vi "SetDAC_04.vi"(0 "RS232/ Optical Fiber":refnum<visa-resource-name>="COM2", 1 "DATA (V)":dbl min=-5000.0 max=5000.0 step=0.001 format="%.2f", 2 "DAC nr":u8=1, 3 "All to zero":bool, 4 "DAC write (mV)":dbl[](array[numeric]) min=-2000.0 max=2000.0) -> (5 "DAC read (mV)":dbl[](array[numeric]))   [LabVIEW 2011]
uses:
  DACreadglobal.vi
panel:
  # "Dilution room :  COM2"
  # "Set dac value manually\nDac values are swept safely"
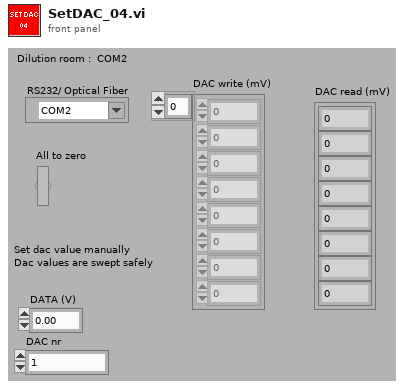
[diagram p1: front panel]
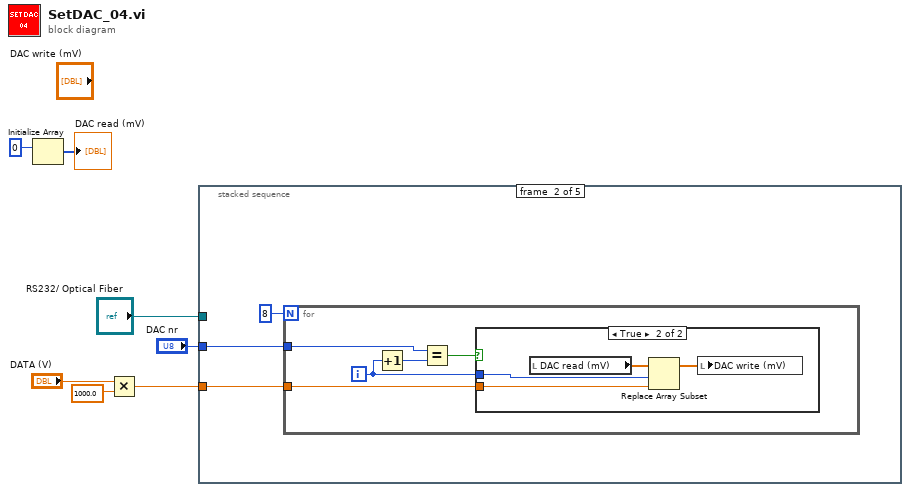
[diagram p0: block diagram]
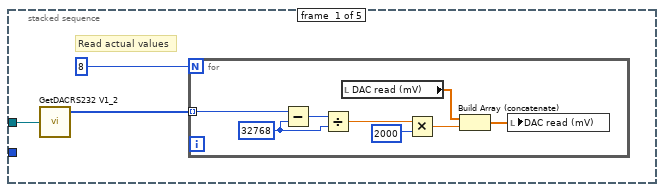
[diagram p2: hidden frame]
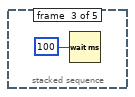
[diagram p4: hidden frame]
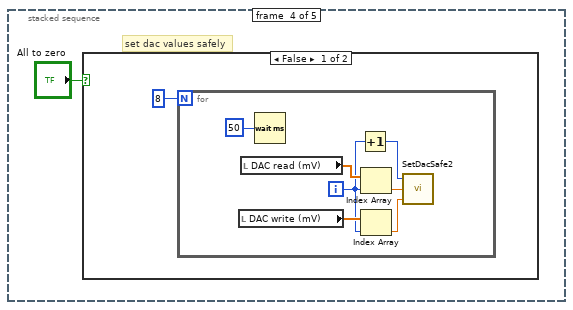
[diagram p5: hidden frame]
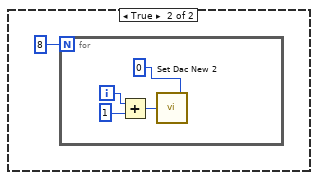
[diagram p6: hidden frame]
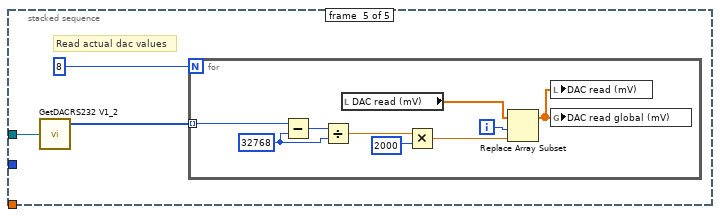
[diagram p7: hidden frame]
diagram:
  n1 = Initialize Array(0) -> (→"DAC read (mV)":i32[])  [unwired: 1 in]
  n2 = Multiply(x="DATA (V)", y=1000.0) -> (x*y=w1:dbl)
  n3 = stacked-sequence {
    tunnel: "RS232/ Optical Fiber" -> [w10 _ _ _ w48]
    tunnel: "DAC nr" -> [_ w20 _ _ _]
    tunnel: w1 -> [_ w19 _ _ _]
    frame #0 {
      # "Read actual values"
      n4 = call "GetDACRS232 V1_2.vi"("VISA resource name IN"=w10) -> ("DAC data out\n(hexadecimaal)"=w8:u16[])  [unwired: 2 in, 2 out]
      n5 = for {
        N: 8 -> [_]
        tunnel: w8 -> [w14] mode=indexing
        w17 = 32768
        n6 = Subtract(x=w14, y=w17) -> (x-y=w18:i32)
        n7 = Divide(x=w18, y=w17) -> (x/y=w16:dbl)
        n8 = local read "DAC read (mV)"() -> (w13:dbl[])
        n9 = Multiply(x=w16, y=2000) -> (x*y=w11:dbl)
        n10 = Build Array (concatenate)(w13, w11) -> (w12:dbl[])
        n11 = local write "DAC read (mV)"(w12) -> ()
      }
    }
    frame #1 {
      n12 = for {
        N: 8 -> [_]
        tunnel: w20 -> [w25]
        tunnel: w19 -> [w22]
        i -> [w23]
        n13 = Increment(x=w23) -> (x+1=w26:i32)
        n14 = Equal?(x=w25, y=w26) -> (x = y?=w24:bool)
        n15 = case shown="True" w24 {
          tunnel: w23 -> [_ w30]
          tunnel: w22 -> [_ w29]
          frame False {
          }
          frame True {
            n16 = local read "DAC read (mV)"() -> (w28:dbl[])
            n17 = Replace Array Subset(array=w28, new element=w29, index=w30) -> (w27:dbl[])
            n18 = local write "DAC write (mV)"(w27) -> ()
          }
        }
      }
    }
    frame #2 {
      n19 = Wait (ms)(milliseconds to wait=100) -> ()  [unwired: 1 out]
    }
    frame #3 {
      # "set dac values safely"
      n20 = case shown="False" "All to zero" {
        frame False {
          n21 = for {
            N: 8 -> [_]
            i -> [w37]
            n22 = local read "DAC write (mV)"() -> (w39:dbl[])
            n23 = local read "DAC read (mV)"() -> (w38:dbl[])
            n24 = Wait (ms)(milliseconds to wait=50) -> ()  [unwired: 1 out]
            n25 = Increment(x=w37) -> (x+1=w40:i32)
            n26 = Index Array(array=w38, index=w37) -> (element=w35:dbl)
            n27 = Index Array(array=w39, index=w37) -> (element=w36:dbl)
            n28 = call "SetDacSafe2.vi"("New Value (mV)"=w36, "Actual Value DAC (mV)"=w35, "DAC Nr."=w40) -> ()  [unwired: 1 out]
          }
        }
        frame True {
          n29 = for {
            N: 8 -> [_]
            i -> [w44]
            n30 = Add(x=w44, y=1) -> (x+y=w43:i32)
            n31 = call "Set Dac New 2.vi"("DATA (V)"=0, "DAC nr"=w43) -> ()
          }
        }
      }
    }
    frame #4 {
      # "Read actual dac values"
      n32 = call "GetDACRS232 V1_2.vi"("VISA resource name IN"=w48) -> ("DAC data out\n(hexadecimaal)"=w46:u16[])  [unwired: 2 in, 2 out]
      n33 = for {
        N: 8 -> [_]
        tunnel: w46 -> [w53] mode=indexing
        i -> [w50]
        w56 = 32768
        n34 = Subtract(x=w53, y=w56) -> (x-y=w57:i32)
        n35 = Divide(x=w57, y=w56) -> (x/y=w55:dbl)
        n36 = local read "DAC read (mV)"() -> (w52:dbl[])
        n37 = Multiply(x=w55, y=2000) -> (x*y=w51:dbl)
        n38 = Replace Array Subset(array=w52, new element=w51, index=w50) -> (w49:dbl[])
        n39 = local write "DAC read (mV)"(w49) -> ()
        n40 = global write "DACreadglobal.vi" "DAC read global (mV)"(w49) -> ()
      }
    }
  }
